vi "KickForceTest.vi"(0 "Game in":refnum<class "Game.lvclass">, 2 "timeout":dbl, 5 "TestParameters":T3, 7 "ballVelocity":dbl, 9 "replace active":bool, 11 "error in (no error)":errorcluster, 12 "grSIM replacement":T4) -> (3 "TestTeam":refnum<class "Ally.lvclass">, 4 "Game out":refnum<class "Game.lvclass">, 6 "replaceRobots":bool, 8 "kickForceTestState":T1={"currentKickForce"=0.0, "targetBallVelocity"=0.0, "est_bal_vell"=0.0, "sample"=0.0, "state"=enum."ReplaceBall"}, 10 "grSIM replacement out":T4, 14 "replaceBall":bool, 15 "error out":errorcluster)   [LabVIEW 2021, in "Game.lvclass"]
uses:
  Game.lvclass
  Controls/grSimReplacement.ctl
  Communication_class/Paths/grSim Packet Command UDP Test Folder/grSim/grSim RobotReplacement.ctl
  Communication_class/Paths/grSim Packet Command UDP Test Folder/grSim/grSim_BallReplacement.ctl
  Ally_class/Ally.lvclass
  D:/RoboIme/horie/SSL_AI/Team_class/Team.lvclass
  Controls/kickForceTestState.ctl
  Controls/KickForceEnum.ctl
  Game.lvclass/Game.ctl
  Team_class/Team.lvclass/Team.ctl
  Ball_class/Ball.lvclass/Ball.ctl
  Object_class/Object.lvclass/Object.ctl
  Robot_class/Robot.lvclass/Robot.ctl
  <vilib>/Analysis/_algsub.llb/Real Vector Norm.vi
  Object_class/Read position(x,y).vi
  Robot_class/Write kick_x.vi
  Robot_class/Write v_tang.vi
  Robot_class/Write dribble.vi
  Read TestTeam.vi
  Read Utilities.lvclass.vi
  Read AllyRef.vi
  Read BallRef.vi
  Read FieldRef.vi
  Ball_class/Read v_x.vi
  Ball_class/Read v_y.vi
  Team_class/Read RobotRef.vi
  Team_class/Write RobotRef.vi
  Ball_class/Ball.lvclass
  D:/RoboIme/horie/SSL_AI/Object_class/Object.lvclass
  Robot_class/Robot.lvclass
  Utilities_class/Utilities.lvclass
  Field_class/Field.lvclass
  <vilib>/Analysis/NI_AALPro.lvlib
panel:
  out "KickForceSTD":dbl[][](array[numeric])
  out "KickForceMean":dbl[][](array[numeric])
  out "kickForceTestList":dbl[][](array[numeric])
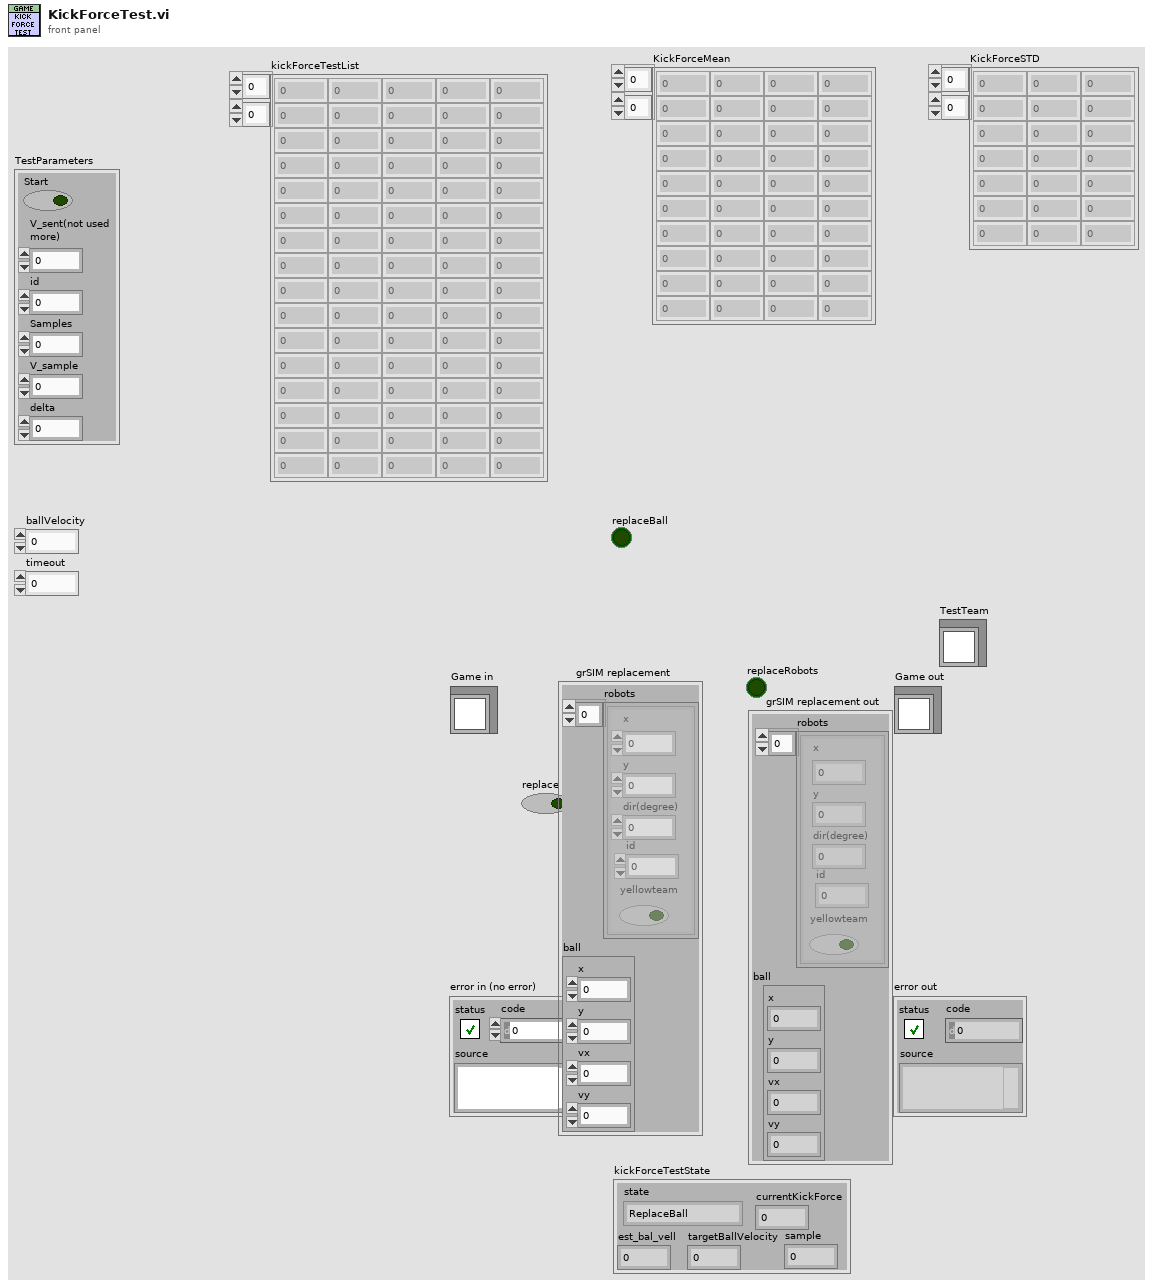
[diagram p1: front panel]
types:
  T1 = typedef "Game.lvclass/kickForceTestState.ctl" = cluster{"currentKickForce":dbl, "targetBallVelocity":dbl, "est_bal_vell":dbl, "sample":dbl, "state":T2}
  T2 = typedef "Game.lvclass/KickForceEnum.ctl" = enum16{"Finish", "Velball", "GoToNextKickForce", "WaitBall", "KickBall", "ReplaceBall"}
  T3 = cluster{"Start":bool, "V_sent(not used\nmore)":dbl, "id":i32, "Samples":dbl, "V_sample":dbl, "delta":dbl}
  T4 = typedef "grSimReplacement.ctl" = cluster{"robots":T5[], "ball":T6}
  T5 = typedef "grSim RobotReplacement.ctl" = cluster{"x":dbl, "y":dbl, "dir(degree)":dbl, "yellowteam":bool, "id":u32}
  T6 = typedef "grSim_BallReplacement.ctl" = cluster{"x":dbl, "y":dbl, "vx":dbl, "vy":dbl}
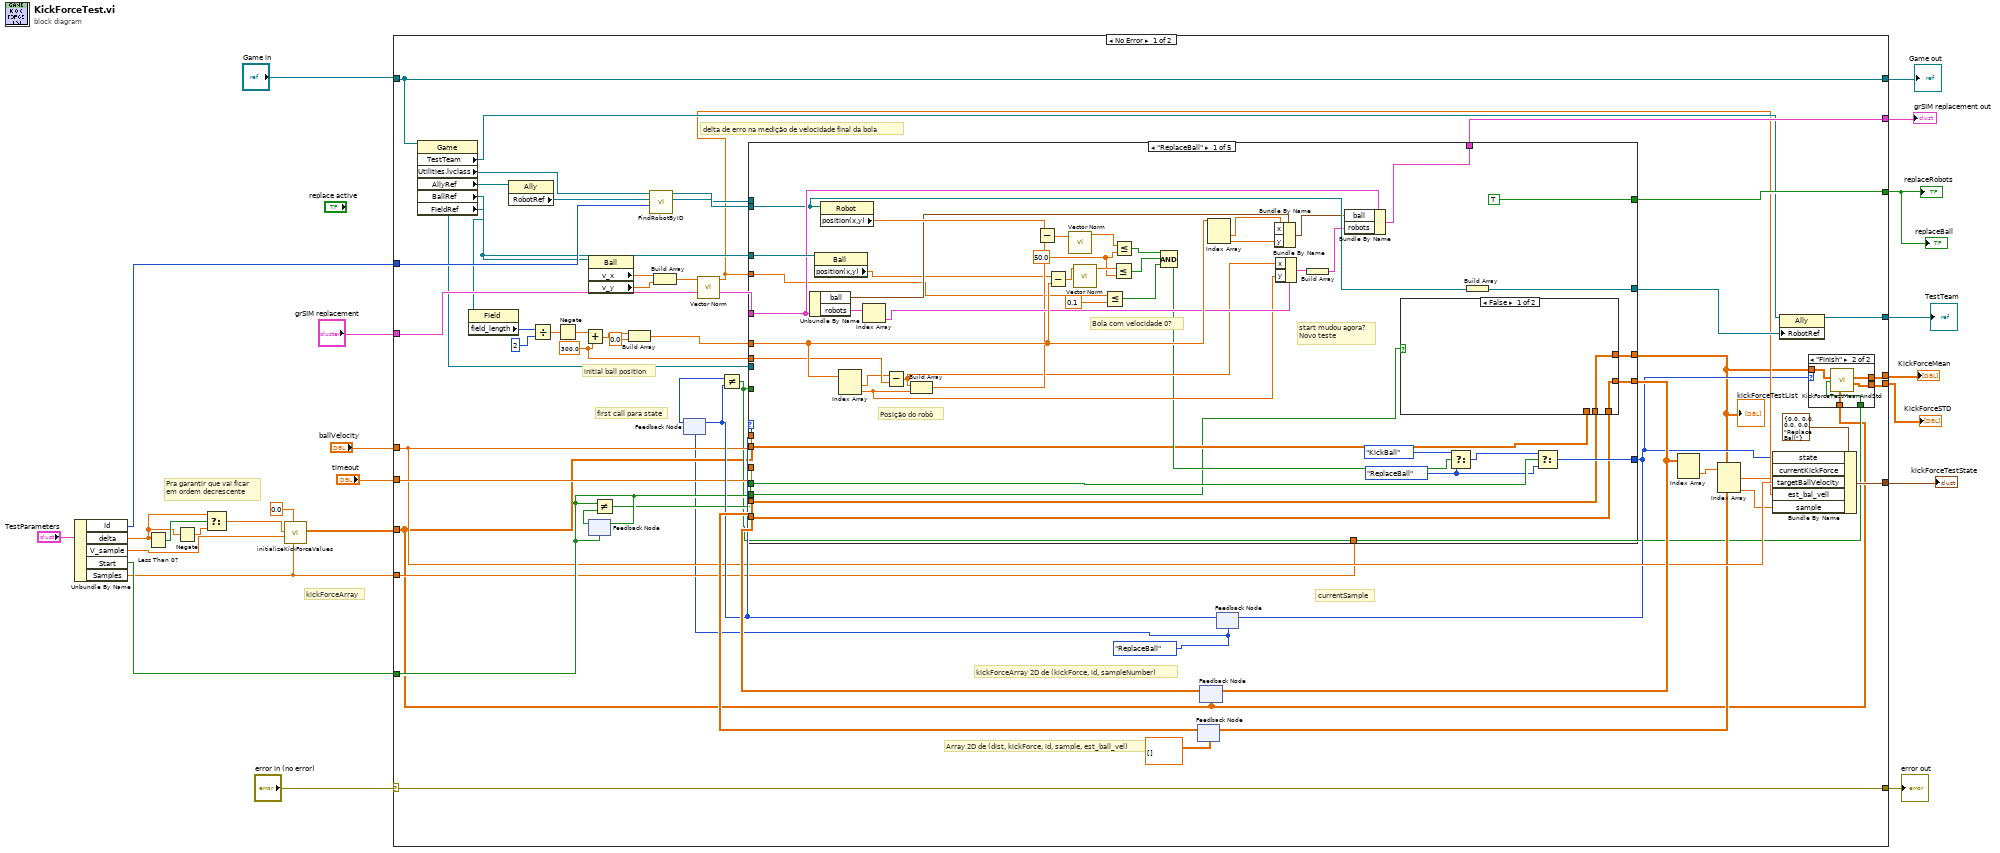
[diagram p0: block diagram]
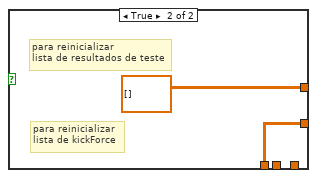
[diagram p3: hidden frame]
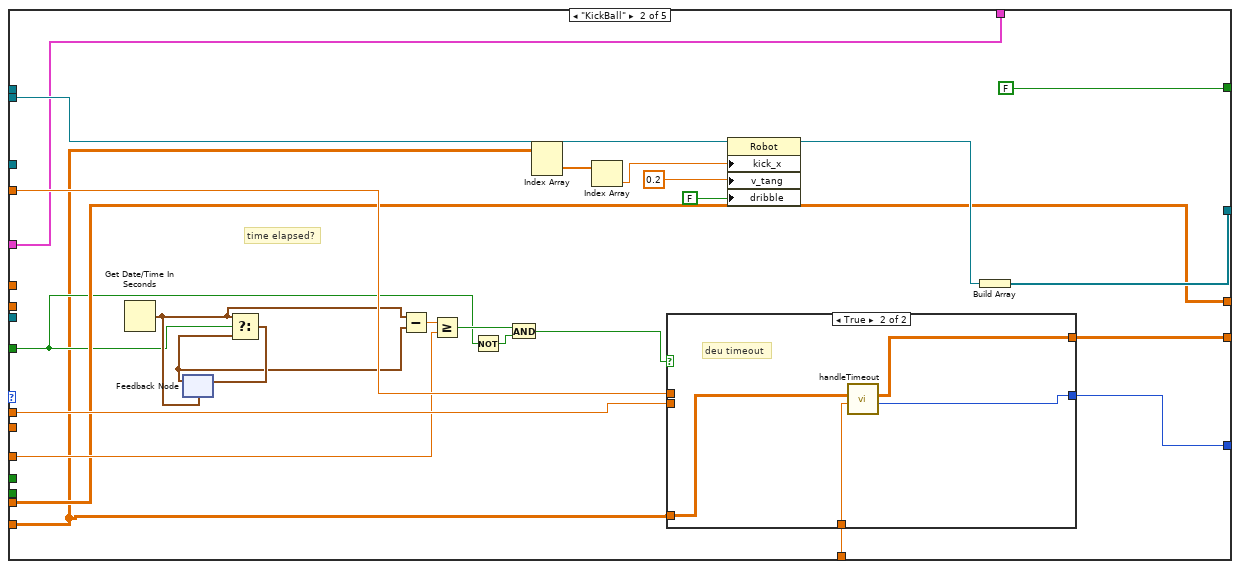
[diagram p4: hidden frame]
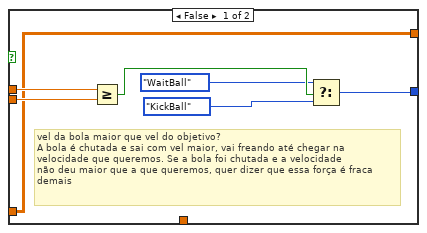
[diagram p5: hidden frame]
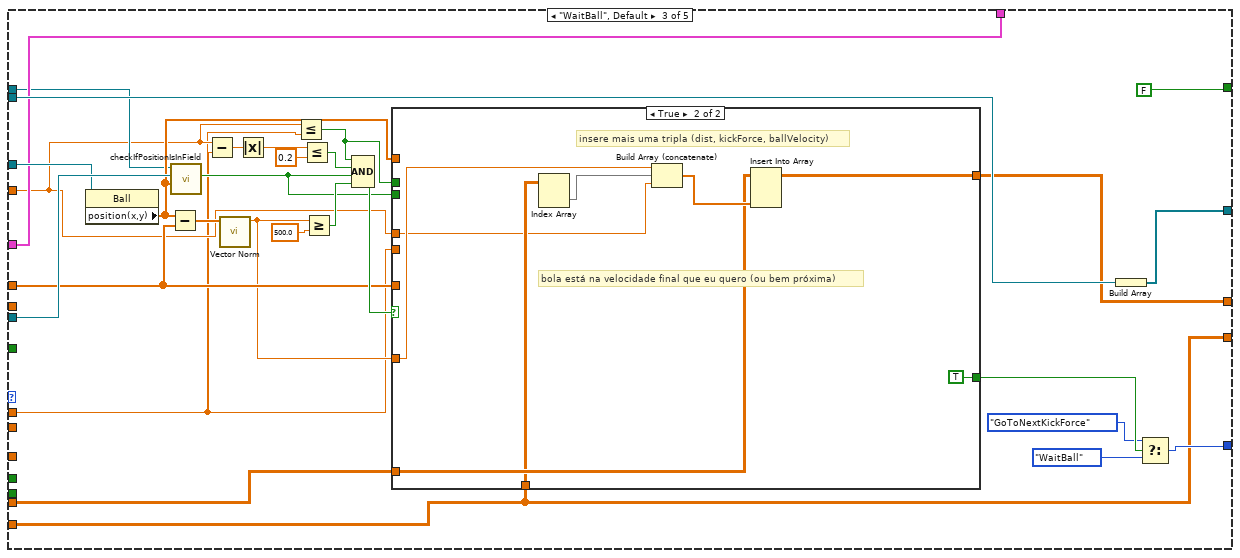
[diagram p6: hidden frame]
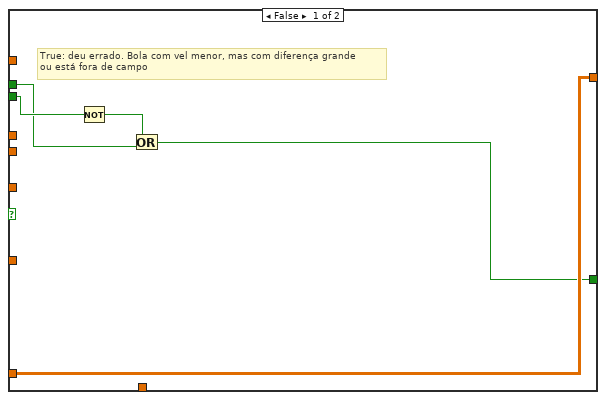
[diagram p7: hidden frame]
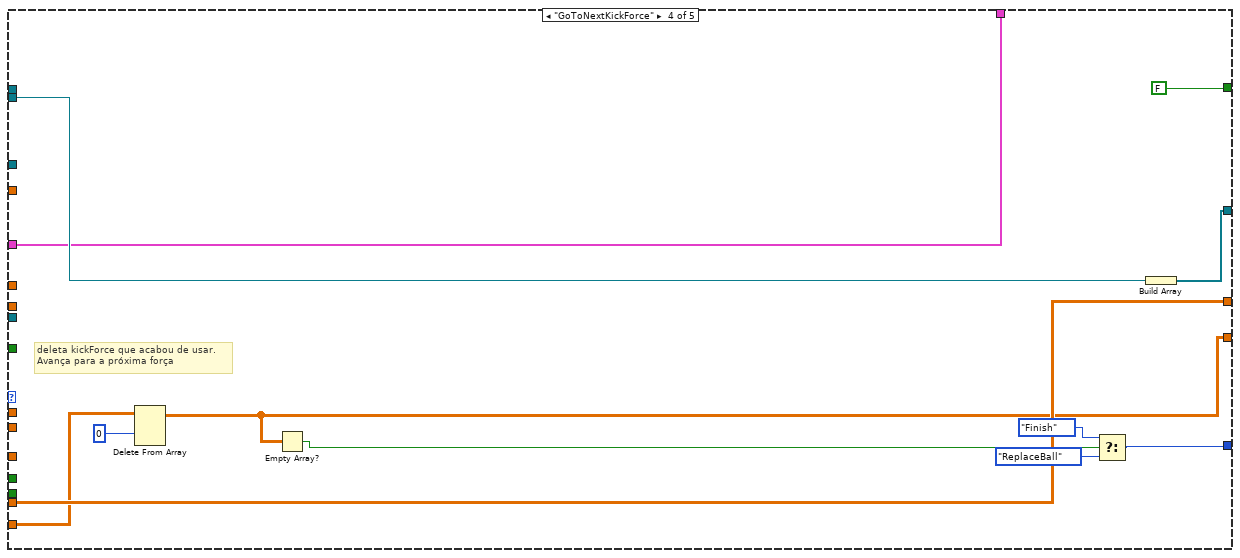
[diagram p8: hidden frame]
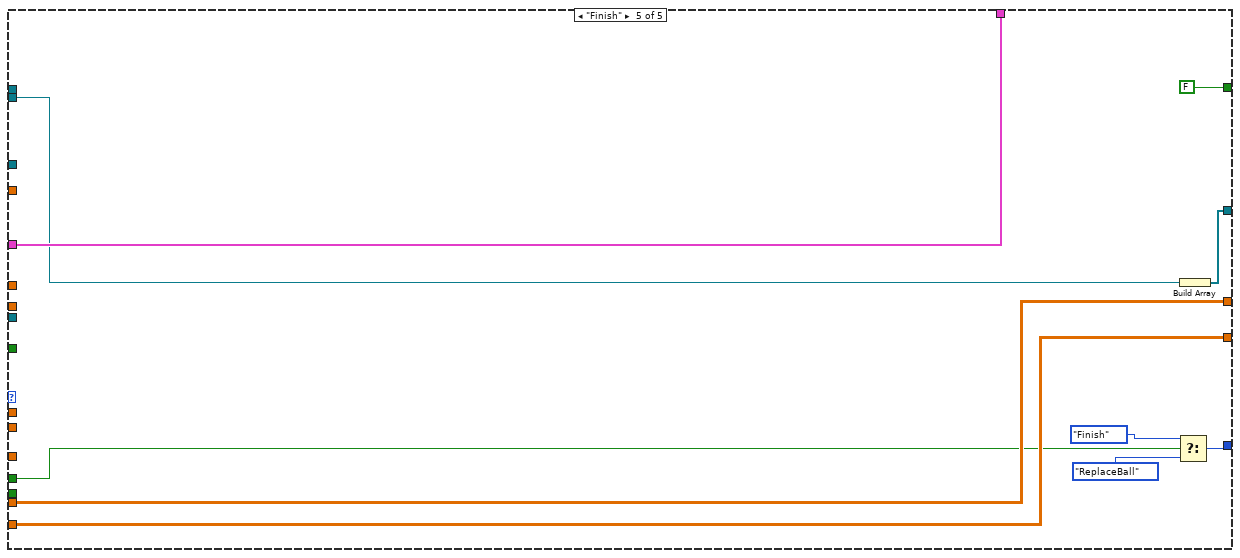
[diagram p9: hidden frame]
diagram:
  # "Pra garantir que vai ficar\nem ordem decrescente"
  # "kickForceArray"
  n1 = Unbundle By Name("TestParameters") -> ("id"=w12:i32, "delta"=w10:dbl, "V_sample"=w7:dbl, "Start"=w13:bool, "Samples"=w6:dbl)
  n2 = Less Than 0?(x=w10) -> (x < 0?=w11:bool)
  n3 = Negate(x=w10) -> (-x=w9:dbl)
  n4 = Select(t=w10, s=w11, f=w9) -> (s? t:f=w8:dbl)
  n5 = call "initializeKickForceValues.vi"("samples"=w6, "kickforce_min"=0.0 ("end"), "kickforce_max"=w7, "delta"=w8) -> ("kickForceList"=w4:dbl[][])  [unwired: 5 in, 2 out]
  n6 = case shown="No Error" "error in (no error)" {
    selector: "error in (no error)" -> [w76 w231]
    tunnel: [w76 w231] -> w23
    tunnel: [w72 w230] -> w21
    tunnel: "Game in" -> [w72 w230]
    tunnel: w12 -> [w69 _]
    tunnel: "grSIM replacement" -> [w65 _]
    tunnel: [w75 _] -> w19
    tunnel: [w73 _] -> w18
    tunnel: [w58 _] -> w17
    tunnel: "ballVelocity" -> [w39 _]
    tunnel: w4 -> [w27 _]
    tunnel: "timeout" -> [w46 _]
    tunnel: w13 -> [w42 _]
    tunnel: [w37 _] -> w1
    tunnel: w6 -> [w34 _]
    tunnel: [w31 _] -> w3
    tunnel: [w30 _] -> w2
    frame No Error {
      w26 = KickForceEnum."ReplaceBall" ("kickForceEnum")
      w56 = 300.0 ("y")
      # "kickForceArray 2D de (kickForce, id, sampleNumber)"
      # "currentSample"
      # "first call para state"
      # "delta de erro na medição de velocidade final da bola"
      # "Array 2D de (dist, kickForce, id, sample, est_ball_vel)"
      # "initial ball position"
      n7 = property class="Game"(reference=w72) -> ("TestTeam"=w45:refnum<class "Ally.lvclass">, "Utilities.lvclass"=w67:refnum<class "Utilities.lvclass">, "AllyRef"=w71:refnum<class "Ally.lvclass">, "BallRef"=w66:refnum<class "Ball.lvclass">, "FieldRef"=w50:refnum<class "Field.lvclass">)  [unwired: 1 in, 2 out]
      n8 = property class="Field"(reference=w50) -> ("field_length"=w64:i32)  [unwired: 1 in, 2 out]
      n9 = property class="Ally"(reference=w71) -> ("RobotRef"=w70:refnum<class "Robot.lvclass">[])  [unwired: 1 in, 2 out]
      n10 = Divide(x=w64, y=2) -> (x/y=w62:dbl)
      n11 = Negate(x=w62) -> (-x=w61:dbl)
      n12 = Add(x=w61, y=w56) -> (x+y=w60:dbl)
      n13 = feedback-in #1(w42) -> ()
      n14 = feedback #1(w42) -> (w43:bool)
      n15 = property class="Ball"(reference=w66) -> ("v_x"=w54:dbl, "v_y"=w55:dbl)  [unwired: 1 in, 2 out]
      n16 = Not Equal?(x=w42, y=w43) -> (x != y?=w41:bool)
      n17 = Build Array(w60, 0.0 ("element")) -> (w57:dbl[])
      n18 = call "FindRobotByID.vi"("id"=w69, "RobotRef"=w70, "Utilities in"=w67) -> ("Robot"=w68:refnum<class "Robot.lvclass">, "Utilities out"=w44:refnum<class "Utilities.lvclass">)  [unwired: 5 in, 2 out]
      n19 = Build Array(w54, w55) -> (w53:dbl[])
      n20 = feedback #2(w26) -> (w48:T2)
      n21 = call-poly <vilib>:"Vector Norm.vi"("Input Vector"=w53) -> ("norm"=w38:dbl)  [unwired: 9 in, 1 out]
      n22 = feedback #3(dbl[][] []) -> (w51:dbl[][])
      n23 = feedback #4(w27) -> (w49:dbl[][])
      n24 = feedback #5(w26) -> (w47:T2)
      n25 = feedback-in #2(w47) -> ()
      n26 = Not Equal?(x=w48, y=w47) -> (x != y?=w28:bool)
      n27 = case shown="\"ReplaceBall\"" w47 {
        tunnel: [w118 w154 w192 w216 w224] -> w74
        tunnel: [TRUE ("replaceRobots") FALSE ("replaceRobots") FALSE ("replaceRobots") FALSE ("replaceRobots") FALSE ("replaceRobots")] -> w73
        tunnel: w68 -> [w119 w149 w193 w215 w225]
        tunnel: w66 -> [w124 _ w183 _ _]
        tunnel: w65 -> [w123 w139 w173 w213 w229]
        tunnel: [w122 w139 w173 w213 w229] -> w58
        tunnel: w57 -> [w121 _ w179 _ _]
        tunnel: w56 -> [w120 _ _ _ _]
        tunnel: [w92 w147 w181 w209 w222] -> w32
        tunnel: w39 -> [_ w148 w169 _ _]
        tunnel: w38 -> [w86 w146 w170 _ _]
        tunnel: w51 -> [w88 w140 w191 w219 w227]
        tunnel: [w117 w140 w190 w219 w227] -> w29
        tunnel: w49 -> [w87 w131 w174 w218 w226]
        tunnel: w50 -> [_ _ w184 _ _]
        tunnel: [w91 w132 w174 w208 w226] -> w40
        tunnel: w28 -> [_ w135 _ _ _]
        tunnel: w46 -> [_ w142 _ _ _]
        tunnel: w42 -> [w94 _ _ _ w223]
        tunnel: w27 -> [w90 _ _ _ _]
        tunnel: w44 -> [_ _ w172 _ _]
        tunnel: w41 -> [w89 _ _ _ _]
        tunnel: w34 -> [_ w130 _ _ _]
        frame "ReplaceBall" {
          w82 = KickForceEnum."ReplaceBall" ("kickForceEnum")
          w96 = 50.0 ("y")
          # "Bola com velocidade 0?"
          # "start mudou agora?\nNovo teste"
          # "Posição do robô"
          n28 = Unbundle By Name(w123) -> ("ball"=w112:T6, "robots"=w116:T5[])
          n29 = property class="Ball"(reference=w124) -> ("position(x,y)"=w99:dbl[])  [unwired: 1 in, 2 out]
          n30 = property class="Robot"(reference=w119) -> ("position(x,y)"=w115:dbl[])  [unwired: 1 in, 2 out]
          n31 = Index Array(array=w121) -> (element #1=w106:dbl, element #2=w102:dbl)  [unwired: 2 in]
          n32 = Index Array(array=w116) -> (element=w110:T5)  [unwired: 1 in]
          n33 = Subtract(x=w106, y=w120) -> (x-y=w103:dbl)
          n34 = Build Array(w103, w102) -> (w105:dbl[])
          n35 = Subtract(x=w115, y=w105) -> (x-y=w114:dbl[])
          n36 = Subtract(x=w99, y=w121) -> (x-y=w98:dbl[])
          n37 = call-poly <vilib>:"Vector Norm.vi"("Input Vector"=w114) -> ("norm"=w113:dbl)  [unwired: 9 in, 1 out]
          n38 = call-poly <vilib>:"Vector Norm.vi"("Input Vector"=w98) -> ("norm"=w97:dbl)  [unwired: 9 in, 1 out]
          n39 = Less Or Equal?(x=w86, y=0.1) -> (x <= y?=w84:bool)
          n40 = Less Or Equal?(x=w97, y=w96) -> (x <= y?=w95:bool)
          n41 = Less Or Equal?(x=w113, y=w96) -> (x <= y?=w101:bool)
          n42 = Compound Arithmetic op=AND(w101, w95, w84) -> (w100:bool)
          n43 = Index Array(array=w121) -> (element #1=w109:dbl, element #2=w104:dbl)  [unwired: 2 in]
          n44 = Bundle By Name(cluster=w112, "x"=w109, "y"=w104) -> (w111:T6)
          n45 = Bundle By Name(cluster=w110, "x"=w103, "y"=w102) -> (w108:T5)
          n46 = Build Array(w108) -> (w107:T5[])
          n47 = Bundle By Name(cluster=w123, "ball"=w111, "robots"=w107) -> (w122:T4)
          n48 = case shown="False" w89 {
            tunnel: [w127 dbl[][] []] -> w117
            tunnel: [w126 w128] -> w91
            tunnel: w90 -> [_ w128]
            tunnel: w88 -> [w127 _]
            tunnel: w87 -> [w126 _]
            frame False {
            }
            frame True {
              # "para reinicializar\nlista de resultados de teste"
              # "para reinicializar\nlista de kickForce"
            }
          }
          n49 = Select(t=KickForceEnum."KickBall" ("kickForceEnum"), s=w100, f=w82) -> (s? t:f=w93:T2)
          n50 = Build Array(w119) -> (w118:refnum<class "Robot.lvclass">[])
          n51 = Select(t=w93, s=w94, f=w82) -> (s? t:f=w92:T2)
        }
        frame "KickBall" {
          # "time elapsed?"
          n52 = Get Date/Time In Seconds() -> (seconds since 1Jan1904=w141:timestamp)
          n53 = feedback #6(w141) -> (w144:timestamp)
          n54 = Select(t=w141, s=w135, f=w144) -> (s? t:f=w145:timestamp)
          n55 = feedback-in #6(w145) -> ()
          n56 = Subtract(x=w141, y=w144) -> (x-y=w143:dbl)
          n57 = Greater Or Equal?(x=w143, y=w142) -> (x >= y?=w138:bool)
          n58 = Not(x=w135) -> (.not. x?=w136:bool)
          n59 = And(x=w138, y=w136) -> (x .and. y?=w137:bool)
          n60 = Index Array(array=w131) -> (element=w134:dbl[])  [unwired: 2 in]
          n61 = Index Array(array=w134) -> (element=w133:dbl)  [unwired: 1 in]
          n62 = case shown="True" w137 {
            tunnel: w148 -> [w161 _]
            tunnel: [w159 w165] -> w147
            tunnel: w146 -> [w158 _]
            tunnel: [w157 w164] -> w132
            tunnel: w131 -> [w157 w163]
            tunnel: w130 -> [_ w162]
            frame False {
              # "vel da bola maior que vel do objetivo?\nA bola é chutada e sai com vel maior, vai freando até chegar na\nvelocidade que queremos. Se a bola foi chutada e a velocidade\nnão deu maior que a que queremos, quer dizer que essa força é fraca\ndemais"
              n63 = Greater Or Equal?(x=w158, y=w161) -> (x >= y?=w160:bool)
              n64 = Select(t=KickForceEnum."WaitBall" ("kickForceEnum"), s=w160, f=KickForceEnum."KickBall" ("kickForceEnum")) -> (s? t:f=w159:T2)
            }
            frame True {
              # "deu timeout"
              n65 = call "handleTimeout.vi"("samples"=w162, "kickForceArray in"=w163) -> ("nextState"=w165:T2, "kickForceArrayWithCurrentSampleDeleted"=w164:dbl[][])  [unwired: 6 in, 2 out]
            }
          }
          n66 = property class="Robot"(reference=w149, "kick_x"=w133, "v_tang"=0.2, "dribble"=FALSE) -> (reference out=w153:refnum<class "Robot.lvclass">)  [unwired: 1 in, 1 out]
          n67 = Build Array(w153) -> (w154:refnum<class "Robot.lvclass">[])
        }
        frame "WaitBall", Default {
          n68 = property class="Ball"(reference=w183) -> ("position(x,y)"=w180:dbl[])  [unwired: 1 in, 2 out]
          n69 = Subtract(x=w180, y=w179) -> (x-y=w178:dbl[])
          n70 = call "checkIfPositionIsInField.vi"("Position"=w180, "FieldRef"=w184, "Utilities in"=w172) -> ("Position Is In Field?"=w171:bool)  [unwired: 4 in, 4 out]
          n71 = Subtract(x=w170, y=w169) -> (x-y=w189:dbl)
          n72 = call-poly <vilib>:"Vector Norm.vi"("Input Vector"=w178) -> ("norm"=w175:dbl)  [unwired: 9 in, 1 out]
          n73 = Absolute Value(x=w189) -> (abs(x)=w188:dbl)
          n74 = Less Or Equal?(x=w170, y=w169) -> (x <= y?=w168:bool)
          n75 = Less Or Equal?(x=w188, y=0.2) -> (x <= y?=w186:bool)
          n76 = Greater Or Equal?(x=w175, y=500.0) -> (x >= y?=w176:bool)
          n77 = Compound Arithmetic op=AND(w168, w186, w171, w176) -> (w185:bool)
          n78 = case shown="True" w185 {
            tunnel: w179 -> [_ _]
            tunnel: w191 -> [w199 w206]
            tunnel: [w199 w205] -> w190
            tunnel: w180 -> [_ _]
            tunnel: w170 -> [_ w200]
            tunnel: w169 -> [_ _]
            tunnel: [w196 TRUE] -> w182
            tunnel: w175 -> [_ w203]
            tunnel: w174 -> [_ w202]
            tunnel: w171 -> [w198 _]
            tunnel: w168 -> [w195 _]
            frame False {
              # "True: deu errado. Bola com vel menor, mas com diferença grande\nou está fora de campo"
              n79 = Not(x=w198) -> (.not. x?=w197:bool)
              n80 = Or(x=w197, y=w195) -> (x .or. y?=w196:bool)
            }
            frame True {
              # "insere mais uma tripla (dist, kickForce, ballVelocity)"
              # "bola está na velocidade final que eu quero (ou bem próxima)"
              n81 = Index Array(array=w202) -> (element=w201:dbl[])  [unwired: 2 in]
              n82 = Build Array (concatenate)(w203, w201, w200) -> (w207:dbl[])
              n83 = Insert Into Array(array=w206, new element=w207) -> (w205:dbl[][])  [unwired: 2 in]
            }
          }
          n84 = Build Array(w193) -> (w192:refnum<class "Robot.lvclass">[])
          n85 = Select(t=KickForceEnum."GoToNextKickForce" ("kickForceEnum"), s=w182, f=KickForceEnum."WaitBall" ("kickForceEnum")) -> (s? t:f=w181:T2)
        }
        frame "GoToNextKickForce" {
          # "deleta kickForce que acabou de usar.\nAvança para a próxima força"
          n86 = Delete From Array(array=w218, index (row)=0 ("index")) -> (array with subset deleted=w208:dbl[][])  [unwired: 2 in, 1 out]
          n87 = Empty Array?(array=w208) -> (empty?=w212:bool)
          n88 = Select(t=KickForceEnum."Finish" ("f"), s=w212, f=KickForceEnum."ReplaceBall") -> (s? t:f=w209:T2)
          n89 = Build Array(w215) -> (w216:refnum<class "Robot.lvclass">[])
        }
        frame "Finish" {
          n90 = Select(t=KickForceEnum."Finish" ("kickForceEnum"), s=w223, f=KickForceEnum."ReplaceBall" ("kickForceEnum")) -> (s? t:f=w222:T2)
          n91 = Build Array(w225) -> (w224:refnum<class "Robot.lvclass">[])
        }
      }
      "kickForceTestList" <- w29
      n92 = feedback-in #3(w29) -> ()
      n93 = feedback-in #4(w40) -> ()
      n94 = feedback-in #5(w32) -> ()
      n95 = Index Array(array=w40) -> (element=w36:dbl[])  [unwired: 2 in]
      n96 = Index Array(array=w36) -> (element #1=w35:dbl, element #3=w33:dbl)  [unwired: 3 in, 1 out]
      n97 = Bundle By Name(cluster=T1 {"currentKickForce"=0.0, "targetBallVelocity"=0.0, "est_bal_vell"=0.0, "sample"=0.0, "state"=enum."ReplaceBall"} ("kickForceTestState"), "state"=w32, "currentKickForce"=w35, "targetBallVelocity"=w39, "est_bal_vell"=w38, "sample"=w33) -> (w37:T1)
      n98 = property class="Ally"(reference=w45, "RobotRef"=w74) -> (reference out=w75:refnum<class "Ally.lvclass">)  [unwired: 1 in, 1 out]
      n99 = case shown="\"Finish\"" w32 {
        tunnel: [_ w81] -> w31
        tunnel: [_ w80] -> w30
        tunnel: w29 -> [_ w79]
        tunnel: w28 -> [_ w78]
        tunnel: w27 -> [_ w77]
        frame Default {
        }
        frame "Finish" {
          n100 = call "KickForceTestMeanAndStd.vi"("InitialKickForce2DArray"=w77, "firstCall"=w78, "ResultKickForce2DArray"=w79) -> ("KickForceSTD"=w80:dbl[][], "KickForceMean"=w81:dbl[][])  [unwired: 5 in, 2 out]
        }
      }
    }
    frame Error {
    }
  }
  "error out" <- w23
  "Game out" <- w21
  "replaceRobots" <- w18
  "grSIM replacement out" <- w17
  "TestTeam" <- w19
  "replaceBall" <- w18
  "KickForceMean" <- w3
  "KickForceSTD" <- w2
  "kickForceTestState" <- w1
